vi "FP_FindElement.vi"(8 "Size as Array":bool[](array[boolean]), 10 "6DOF telegram":string, 11 "Start position":i32) -> (0 "End position + 1":i32, 3 "Value":u8[](array[numeric]))   [LabVIEW 2013]
panel:
  out "Bytes":i32
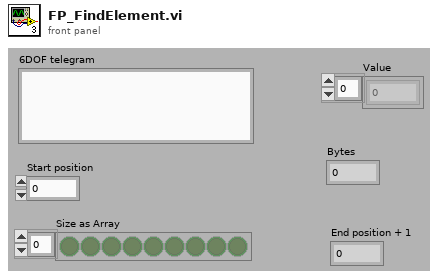
[diagram p1: front panel]
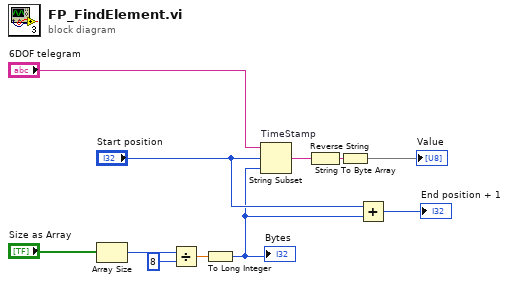
[diagram p0: block diagram]
diagram:
  n1 = Array Size(array="Size as Array") -> (size(s)=w9:i32)
  n2 = Divide(x=w9, y=8) -> (x/y=w7:dbl)
  n3 = To Long Integer(number=w7) -> (32bit integer=w2:i32)
  "Bytes" <- w2
  n4 = String Subset "TimeStamp"(string="6DOF telegram", offset (0)="Start position", length (rest)=w2) -> (substring=w10:string)
  n5 = Reverse String(1:w10) -> (0:w11:string)
  n6 = String To Byte Array(string=w11) -> (unsigned byte array=→"Value":u8[])
  n7 = Add(x="Start position", y=w2) -> (x+y=→"End position + 1":i32)
